vi "Scanner_Ansteuerung_Main.vi"(8 "error in":errorcluster, 10 "Scanner Out-Ports":T1, 11 "Scanner Properties":T2) -> (0 "error out":errorcluster)   [LabVIEW 2009]
uses:
  <vilib>/DAQmx/write.llb/DAQmx Write (Analog 2D DBL NChan NSamp).vi
  <vilib>/DAQmx/configure/timing.llb/DAQmx Timing (Sample Clock).vi
  <vilib>/DAQmx/create/channels.llb/DAQmx Create Channel (AO-Voltage-Basic).vi
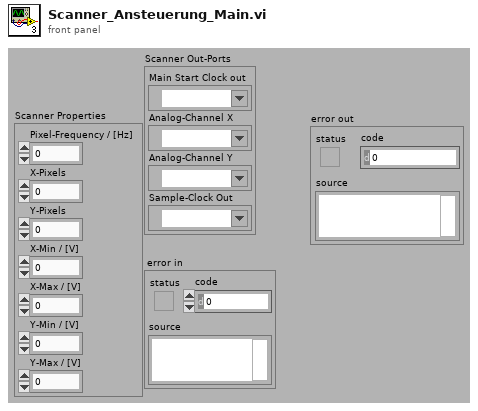
[diagram p1: front panel]
types:
  T1 = cluster{"Main Start Clock out":tag, "Analog-Channel X":tag, "Analog-Channel Y":tag, "Sample-Clock Out":tag}
  T2 = cluster{"Pixel-Frequency / [Hz]":dbl, "X-Pixels":u32, "Y-Pixels":u32, "X-Min / [V]":dbl, "X-Max / [V]":dbl, "Y-Min / [V]":dbl, "Y-Max / [V]":dbl}
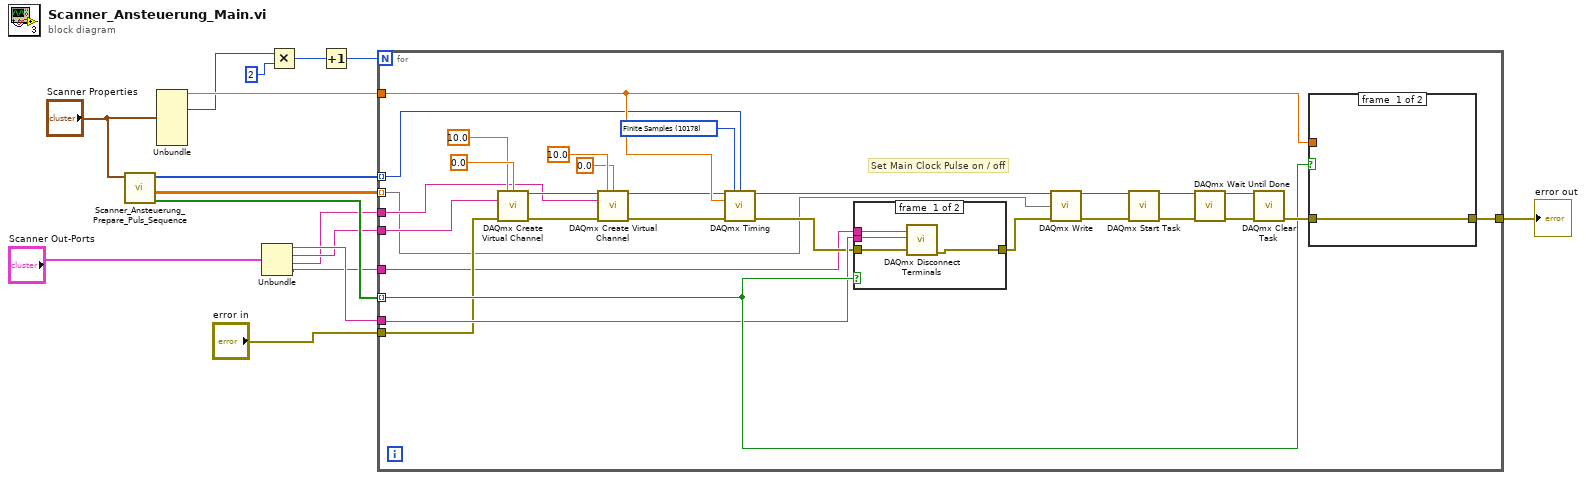
[diagram p0: block diagram]
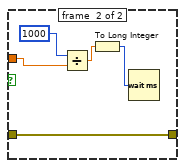
[diagram p2: hidden frame]
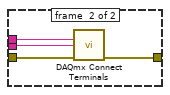
[diagram p3: hidden frame]
diagram:
  n1 = call "Scanner_Ansteuerung_Prepare_Puls_Sequence.vi"("cluster"="Scanner Properties") -> ("Sync-Pulse-Array"=w10:bool[], "Power-Array"=w11:dbl[][][], "Clock-Array"=w12:i32[])  [unwired: 8 out]
  n2 = Unbundle("Scanner Properties") -> ("Pixel-Frequency / [Hz]"=w9:dbl, "Y-Pixels"=w5:u32)  [unwired: 5 out]
  n3 = Unbundle("Scanner Out-Ports") -> ("Main Start Clock out"=w8:tag, "Analog-Channel X"=w7:tag, "Analog-Channel Y"=w6:tag, "Sample-Clock Out"=w2:tag)
  n4 = Multiply(x=w5, y=u32 2) -> (x*y=w14:u32)
  n5 = Increment(x=w14) -> (x+1=w13:u32)
  n6 = for {
    N: w13 -> [_]
    tunnel: w9 -> [w45]
    tunnel: [w44] -> w16
    tunnel: w11 -> [w18] mode=indexing
    tunnel: w12 -> [w28] mode=indexing
    tunnel: w10 -> [w29] mode=indexing
    tunnel: w7 -> [w27]
    tunnel: w6 -> [w26]
    tunnel: w8 -> [w25]
    tunnel: "error in" -> [w24]
    tunnel: w2 -> [w17]
    w43 = 10178 items=["Finite Samples"=10178, "Continuous Samples"=10123, "Hardware Timed Single Point"=12522] ("sample mode")
    # "Set Main Clock Pulse on / off"
    n7 = call-poly <vilib>:"DAQmx Create Virtual Channel.vi"("maximum value"=10.0, "minimum value"=0.0, "physical channels"=w27, "error in"=w24) -> ("task out"=w35:refnum<k21>, "error out"=w36:errorcluster)  [unwired: 5 in, 5 out]
    n8 = call-poly <vilib>:"DAQmx Create Virtual Channel.vi"("task in"=w35, "maximum value"=10.0, "minimum value"=0.0, "physical channels"=w26, "error in"=w36) -> ("task out"=w33:refnum<k21>, "error out"=w34:errorcluster)  [unwired: 4 in, 5 out]
    n9 = call-poly <vilib>:"DAQmx Timing.vi"("task/channels in"=w33, "sample mode"=w43, "samples per channel"=w28, "rate"=w45, "error in"=w34) -> ("task out"=w19:refnum<k21>, "error out"=w23:errorcluster)  [unwired: 2 in, 7 out]
    n10 = case shown="False" w29 {
      tunnel: w25 -> [w54 w59]
      tunnel: w17 -> [w55 w58]
      tunnel: [w52 w56] -> w21
      tunnel: w23 -> [w53 w57]
      frame #0 {
        n11 = call <vilib>:"DAQmx Disconnect Terminals.vi"("source terminal"=w55, "destination terminal"=w54, "error in"=w53) -> ("error out"=w52:errorcluster)  [unwired: 12 out]
      }
      frame #1 {
        n12 = call <vilib>:"DAQmx Connect Terminals.vi"("source terminal"=w58, "destination terminal"=w59, "error in"=w57) -> ("error out"=w56:errorcluster)  [unwired: 1 in, 11 out]
      }
    }
    n13 = call-poly <vilib>:"DAQmx Write.vi"("task/channels in"=w19, "data"=w18, "error in"=w21) -> ("task out"=w22:refnum<k21>, "error out"=w20:errorcluster)  [unwired: 1 in, 10 out]
    n14 = call <vilib>:"DAQmx Start Task.vi"("task/channels in"=w22, "error in"=w20) -> ("task out"=w30:refnum<k21>, "error out"=w31:errorcluster)  [unwired: 12 out]
    n15 = call <vilib>:"DAQmx Wait Until Done.vi"("task/channels in"=w30, "error in"=w31) -> ("task out"=w42:refnum<k21>, "error out"=w41:errorcluster)  [unwired: 1 in, 11 out]
    n16 = call <vilib>:"DAQmx Clear Task.vi"("task in"=w42, "error in"=w41) -> ("error out"=w32:errorcluster)  [unwired: 13 out]
    n17 = case shown="True" w29 {
      tunnel: w32 -> [w46 w51]
      tunnel: [w46 w51] -> w44
      tunnel: w45 -> [_ w49]
      frame #0 {
      }
      frame #1 {
        n18 = Divide(x=1000, y=w49) -> (x/y=w48:dbl)
        n19 = To Long Integer(number=w48) -> (32bit integer=w47:i32)
        n20 = Wait (ms)(milliseconds to wait=w47) -> ()  [unwired: 1 out]
      }
    }
  }
  "error out" <- w16
